vi "enable_all_controls.vi"(0 "input cluster":T1) -> ()   [LabVIEW 2010]
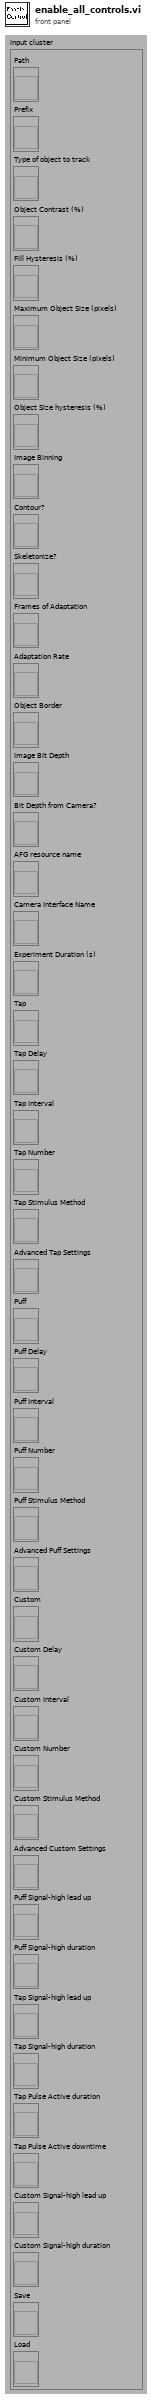
[diagram p1: front panel]
types:
  T1 = cluster{"Path":refnum<vi>, "Prefix":refnum<vi>, "Type of object to track":refnum<vi>, "Object Contrast (%)":refnum<vi>, "Fill Hysteresis (%)":refnum<vi>, "Maximum Object Size (pixels)":refnum<vi>, "Minimum Object Size (pixels)":refnum<vi>, "Object Size hysteresis (%)":refnum<vi>, "Image Binning":refnum<vi>, "Contour?":refnum<vi>, "Skeletonize?":refnum<vi>, "Frames of Adaptation":refnum<vi>, "Adaptation Rate":refnum<vi>, "Object Border":refnum<vi>, "Image Bit Depth":refnum<vi>, "Bit Depth from Camera?":refnum<vi>, "AFG resource name":refnum<vi>, "Camera Interface Name":refnum<vi>, "Experiment Duration (s)":refnum<vi>, "Tap":refnum<vi>, "Tap Delay":refnum<vi>, "Tap Interval":refnum<vi>, "Tap Number":refnum<vi>, "Tap Stimulus Method":refnum<vi>, "Advanced Tap Settings":refnum<vi>, "Puff":refnum<vi>, "Puff Delay":refnum<vi>, "Puff Interval":refnum<vi>, "Puff Number":refnum<vi>, "Puff Stimulus Method":refnum<vi>, "Advanced Puff Settings":refnum<vi>, "Custom":refnum<vi>, "Custom Delay":refnum<vi>, "Custom Interval":refnum<vi>, "Custom Number":refnum<vi>, "Custom Stimulus Method":refnum<vi>, "Advanced Custom Settings":refnum<vi>, "Puff Signal-high lead up":refnum<vi>, "Puff Signal-high duration":refnum<vi>, "Tap Signal-high lead up":refnum<vi>, "Tap Signal-high duration":refnum<vi>, "Tap Pulse Active duration":refnum<vi>, "Tap Pulse Active downtime":refnum<vi>, "Custom Signal-high lead up":refnum<vi>, "Custom Signal-high duration":refnum<vi>, "Save":refnum<vi>, "Load":refnum<vi>}
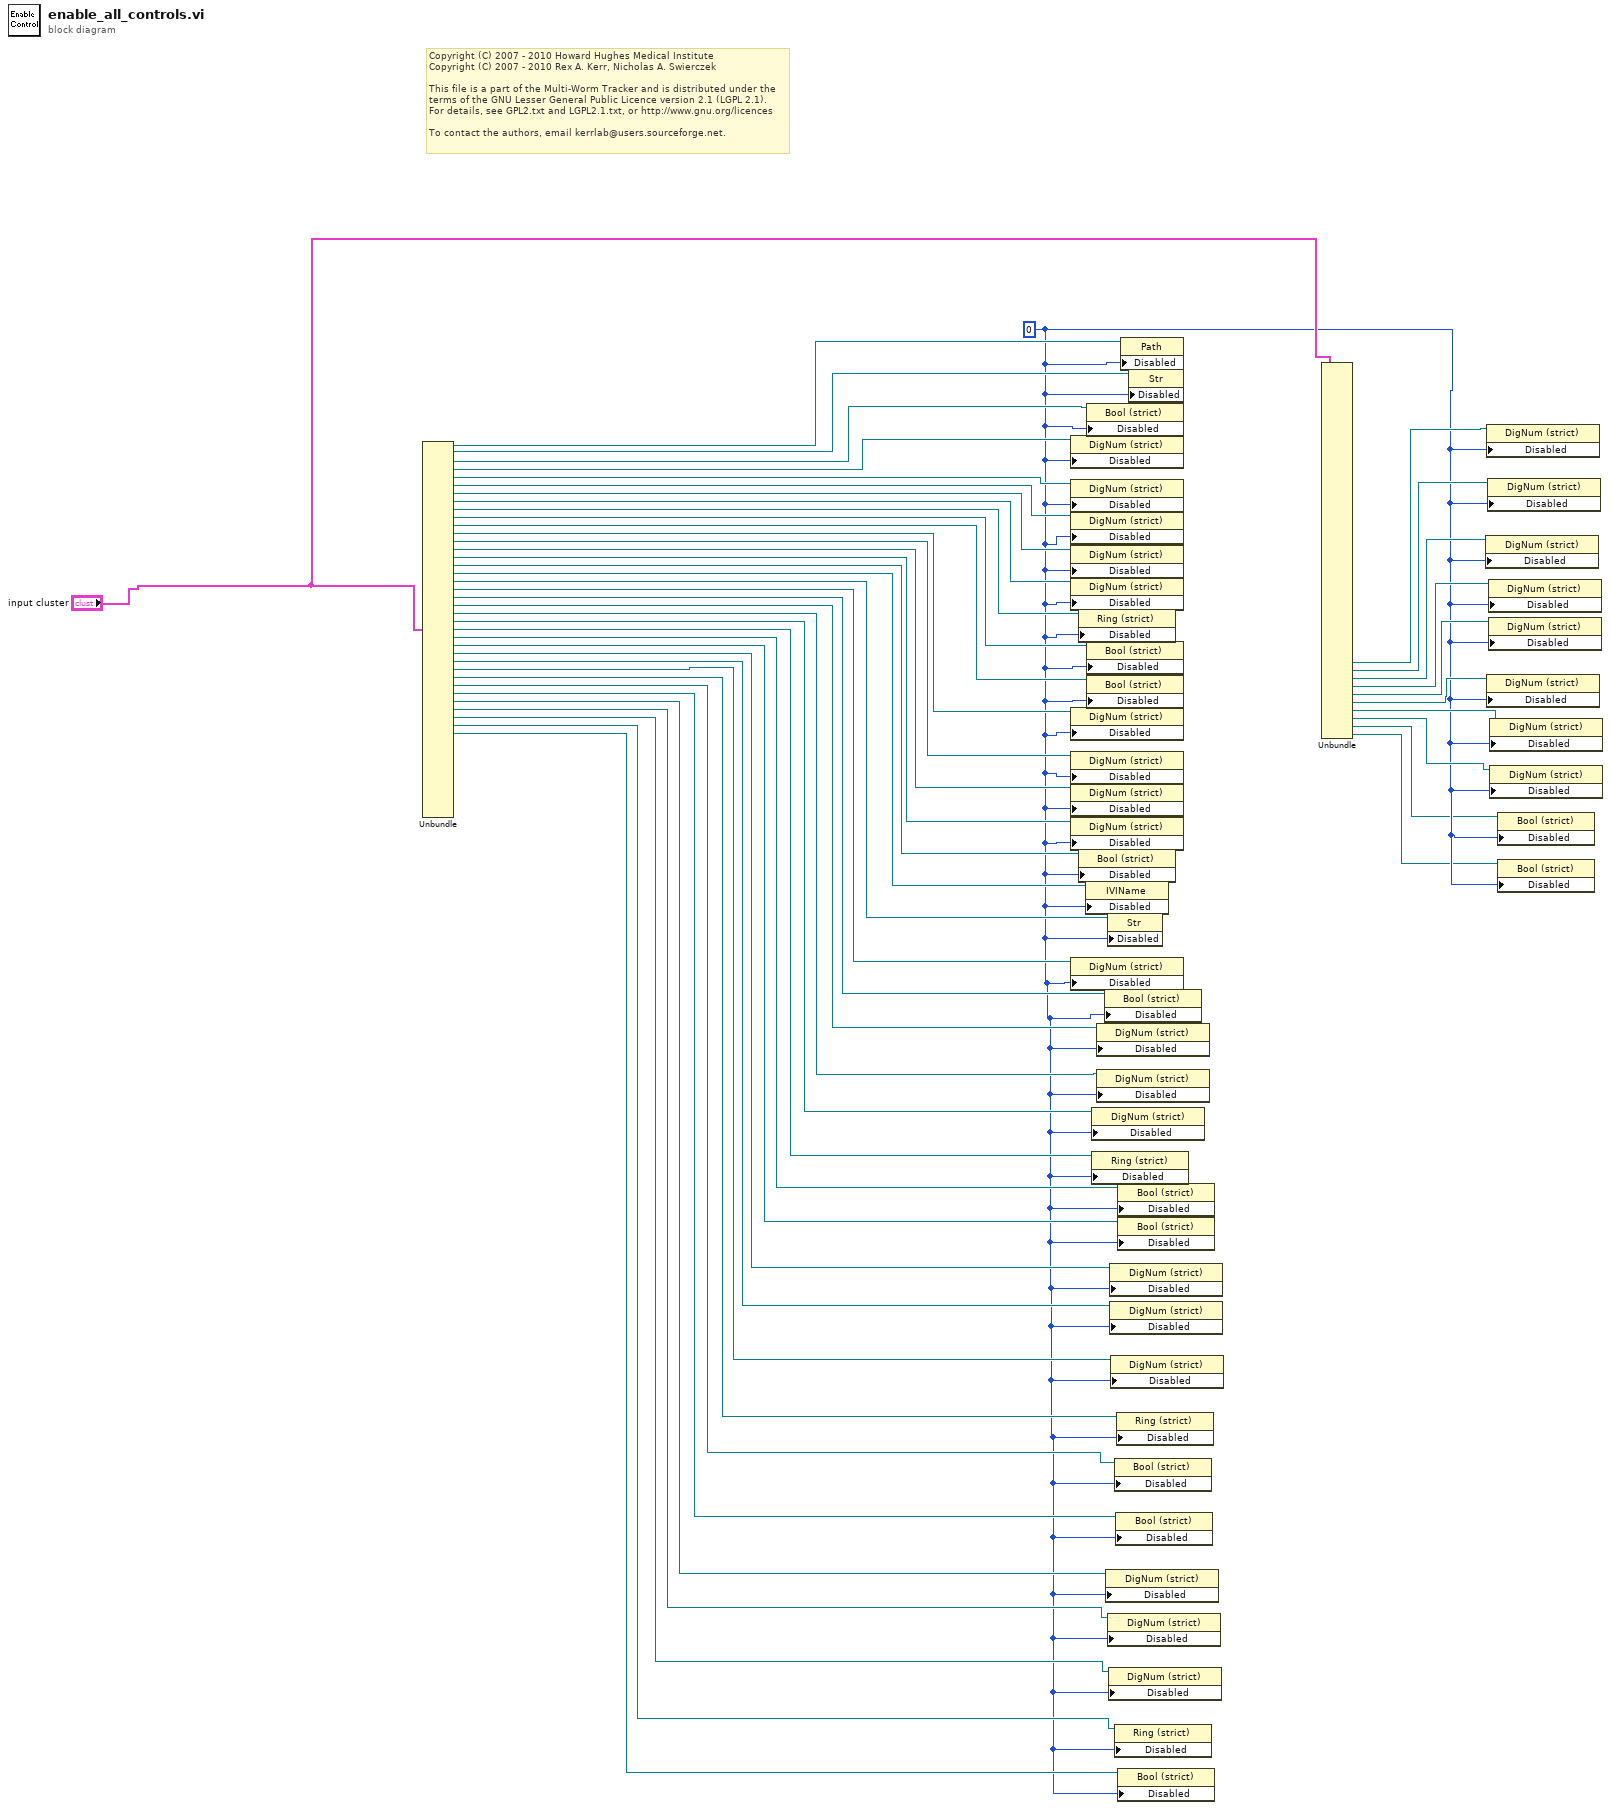
[diagram p0: block diagram]
diagram:
  w3 = u8 0
  # "Copyright (C) 2007 - 2010 Howard Hughes Medical Institute\nCopyright (C) 2007 - 2010 Rex A. Kerr, Nicholas A. Swierczek\n \nThis file is a part of the Multi-Worm Tracker and is distributed under the\nterms of the GNU Lesser General Public Licence version 2.1 (LGPL 2.1).\nFor details, see GPL2.txt and LGPL2.1.txt, or http://www.gnu.org/licences\n \nTo contact the authors, email kerrlab@users.sourceforge.net."
  n1 = Unbundle("input cluster") -> ("Path"=w49:refnum<vi>, "Prefix"=w48:refnum<vi>, "Type of object to track"=w47:refnum<vi>, "Object Contrast (%)"=w46:refnum<vi>, "Fill Hysteresis (%)"=w45:refnum<vi>, "Maximum Object Size (pixels)"=w44:refnum<vi>, "Minimum Object Size (pixels)"=w43:refnum<vi>, "Object Size hysteresis (%)"=w42:refnum<vi>, "Image Binning"=w41:refnum<vi>, "Contour?"=w40:refnum<vi>, "Skeletonize?"=w39:refnum<vi>, "Frames of Adaptation"=w38:refnum<vi>, "Adaptation Rate"=w37:refnum<vi>, "Object Border"=w36:refnum<vi>, "Image Bit Depth"=w35:refnum<vi>, "Bit Depth from Camera?"=w34:refnum<vi>, "AFG resource name"=w33:refnum<vi>, "Camera Interface Name"=w32:refnum<vi>, "Experiment Duration (s)"=w31:refnum<vi>, "Tap"=w30:refnum<vi>, "Tap Delay"=w29:refnum<vi>, "Tap Interval"=w28:refnum<vi>, "Tap Number"=w27:refnum<vi>, "Tap Stimulus Method"=w26:refnum<vi>, "Advanced Tap Settings"=w25:refnum<vi>, "Puff"=w24:refnum<vi>, "Puff Delay"=w23:refnum<vi>, "Puff Interval"=w22:refnum<vi>, "Puff Number"=w21:refnum<vi>, "Puff Stimulus Method"=w20:refnum<vi>, "Advanced Puff Settings"=w19:refnum<vi>, "Custom"=w18:refnum<vi>, "Custom Delay"=w17:refnum<vi>, "Custom Interval"=w16:refnum<vi>, "Custom Number"=w15:refnum<vi>, "Custom Stimulus Method"=w14:refnum<vi>, "Advanced Custom Settings"=w13:refnum<vi>)  [unwired: 10 out]
  n2 = property class="DigNum (strict)"(reference=w46, "Disabled"=w3) -> ()  [unwired: 1 in, 2 out]
  n3 = property class="DigNum (strict)"(reference=w45, "Disabled"=w3) -> ()  [unwired: 1 in, 2 out]
  n4 = property class="DigNum (strict)"(reference=w44, "Disabled"=w3) -> ()  [unwired: 1 in, 2 out]
  n5 = property class="DigNum (strict)"(reference=w43, "Disabled"=w3) -> ()  [unwired: 1 in, 2 out]
  n6 = property class="DigNum (strict)"(reference=w42, "Disabled"=w3) -> ()  [unwired: 1 in, 2 out]
  n7 = property class="DigNum (strict)"(reference=w38, "Disabled"=w3) -> ()  [unwired: 1 in, 2 out]
  n8 = property class="DigNum (strict)"(reference=w37, "Disabled"=w3) -> ()  [unwired: 1 in, 2 out]
  n9 = property class="DigNum (strict)"(reference=w36, "Disabled"=w3) -> ()  [unwired: 1 in, 2 out]
  n10 = property class="DigNum (strict)"(reference=w35, "Disabled"=w3) -> ()  [unwired: 1 in, 2 out]
  n11 = property class="DigNum (strict)"(reference=w31, "Disabled"=w3) -> ()  [unwired: 1 in, 2 out]
  n12 = property class="Ring (strict)"(reference=w41, "Disabled"=w3) -> ()  [unwired: 1 in, 2 out]
  n13 = property class="Bool (strict)"(reference=w34, "Disabled"=w3) -> ()  [unwired: 1 in, 2 out]
  n14 = property class="IVIName"(reference=w33, "Disabled"=w3) -> ()  [unwired: 1 in, 2 out]
  n15 = property class="Bool (strict)"(reference=w47, "Disabled"=w3) -> ()  [unwired: 1 in, 2 out]
  n16 = property class="Bool (strict)"(reference=w40, "Disabled"=w3) -> ()  [unwired: 1 in, 2 out]
  n17 = property class="Bool (strict)"(reference=w39, "Disabled"=w3) -> ()  [unwired: 1 in, 2 out]
  n18 = property class="DigNum (strict)"(reference=w27, "Disabled"=w3) -> ()  [unwired: 1 in, 2 out]
  n19 = property class="Ring (strict)"(reference=w26, "Disabled"=w3) -> ()  [unwired: 1 in, 2 out]
  n20 = property class="DigNum (strict)"(reference=w29, "Disabled"=w3) -> ()  [unwired: 1 in, 2 out]
  n21 = property class="DigNum (strict)"(reference=w28, "Disabled"=w3) -> ()  [unwired: 1 in, 2 out]
  n22 = property class="Bool (strict)"(reference=w30, "Disabled"=w3) -> ()  [unwired: 1 in, 2 out]
  n23 = property class="DigNum (strict)"(reference=w17, "Disabled"=w3) -> ()  [unwired: 1 in, 2 out]
  n24 = property class="Str"(reference=w32, "Disabled"=w3) -> ()  [unwired: 1 in, 2 out]
  n25 = property class="DigNum (strict)"(reference=w16, "Disabled"=w3) -> ()  [unwired: 1 in, 2 out]
  n26 = property class="DigNum (strict)"(reference=w15, "Disabled"=w3) -> ()  [unwired: 1 in, 2 out]
  n27 = property class="DigNum (strict)"(reference=w23, "Disabled"=w3) -> ()  [unwired: 1 in, 2 out]
  n28 = property class="DigNum (strict)"(reference=w22, "Disabled"=w3) -> ()  [unwired: 1 in, 2 out]
  n29 = property class="DigNum (strict)"(reference=w21, "Disabled"=w3) -> ()  [unwired: 1 in, 2 out]
  n30 = property class="Bool (strict)"(reference=w19, "Disabled"=w3) -> ()  [unwired: 1 in, 2 out]
  n31 = property class="Ring (strict)"(reference=w14, "Disabled"=w3) -> ()  [unwired: 1 in, 2 out]
  n32 = property class="Bool (strict)"(reference=w18, "Disabled"=w3) -> ()  [unwired: 1 in, 2 out]
  n33 = property class="Ring (strict)"(reference=w20, "Disabled"=w3) -> ()  [unwired: 1 in, 2 out]
  n34 = property class="Bool (strict)"(reference=w25, "Disabled"=w3) -> ()  [unwired: 1 in, 2 out]
  n35 = property class="Bool (strict)"(reference=w24, "Disabled"=w3) -> ()  [unwired: 1 in, 2 out]
  n36 = property class="Bool (strict)"(reference=w13, "Disabled"=w3) -> ()  [unwired: 1 in, 2 out]
  n37 = property class="Path"(reference=w49, "Disabled"=w3) -> ()  [unwired: 1 in, 2 out]
  n38 = property class="Str"(reference=w48, "Disabled"=w3) -> ()  [unwired: 1 in, 2 out]
  n39 = Unbundle("input cluster") -> ("Puff Signal-high lead up"=w12:refnum<vi>, "Puff Signal-high duration"=w11:refnum<vi>, "Tap Signal-high lead up"=w10:refnum<vi>, "Tap Signal-high duration"=w9:refnum<vi>, "Tap Pulse Active duration"=w8:refnum<vi>, "Tap Pulse Active downtime"=w7:refnum<vi>, "Custom Signal-high lead up"=w6:refnum<vi>, "Custom Signal-high duration"=w5:refnum<vi>, "Save"=w2:refnum<vi>, "Load"=w1:refnum<vi>)  [unwired: 37 out]
  n40 = property class="DigNum (strict)"(reference=w10, "Disabled"=w3) -> ()  [unwired: 1 in, 2 out]
  n41 = property class="DigNum (strict)"(reference=w12, "Disabled"=w3) -> ()  [unwired: 1 in, 2 out]
  n42 = property class="DigNum (strict)"(reference=w7, "Disabled"=w3) -> ()  [unwired: 1 in, 2 out]
  n43 = property class="DigNum (strict)"(reference=w11, "Disabled"=w3) -> ()  [unwired: 1 in, 2 out]
  n44 = property class="DigNum (strict)"(reference=w9, "Disabled"=w3) -> ()  [unwired: 1 in, 2 out]
  n45 = property class="DigNum (strict)"(reference=w8, "Disabled"=w3) -> ()  [unwired: 1 in, 2 out]
  n46 = property class="DigNum (strict)"(reference=w6, "Disabled"=w3) -> ()  [unwired: 1 in, 2 out]
  n47 = property class="DigNum (strict)"(reference=w5, "Disabled"=w3) -> ()  [unwired: 1 in, 2 out]
  n48 = property class="Bool (strict)"(reference=w2, "Disabled"=w3) -> ()  [unwired: 1 in, 2 out]
  n49 = property class="Bool (strict)"(reference=w1, "Disabled"=w3) -> ()  [unwired: 1 in, 2 out]
